vi "Slaver.vi"() -> ()   [LabVIEW 2014]
panel:
  out "에러 출력":errorcluster
  out "웨이브폼 그래프":dbl[](graph)
  in  "정지":bool
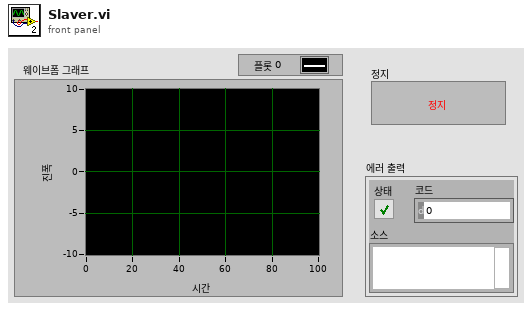
[diagram p1: front panel]
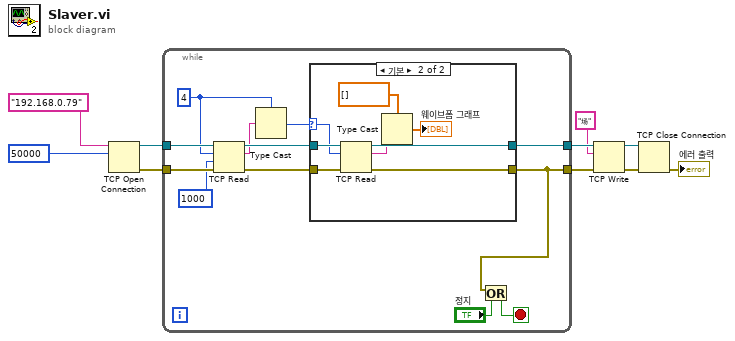
[diagram p0: block diagram]
diagram:
  n1 = TCP Open Connection(address="192.168.0.79" ("주소"), remote port or service name=u16 50000 ("원격 포트 또는 서비스 이름")) -> (connection ID=w8:refnum<k5>, error out=w7:errorcluster)  [unwired: 3 in]
  n2 = while {
    tunnel: w8 -> [w22]
    tunnel: [w20] -> w4
    tunnel: w7 -> [w19]
    tunnel: [w12] -> w3
    stop <- w13 stop-if-true
    w16 = 4 ("읽을 바이트")
    n3 = TCP Read(connection ID=w22, bytes to read=w16, error in (no error)=w19, 9:1000 ("타임아웃 ms (25000)")) -> (connection ID out=w21:refnum<k5>, data out=w17:string, error out=w15:errorcluster)  [unwired: 1 in]
    n4 = Type Cast(type=w16, x=w17) -> (*(type *) &x=w14:i32)
    n5 = case shown="기본" w14 {
      selector: w14 -> [_ w28]
      tunnel: w21 -> [w24 w32]
      tunnel: [w24 w31] -> w20
      tunnel: w15 -> [w23 w30]
      tunnel: [w23 w29] -> w12
      frame ..0 {
      }
      frame Default {
        n6 = TCP Read(connection ID=w32, bytes to read=w28, error in (no error)=w30) -> (connection ID out=w31:refnum<k5>, data out=w27:string, error out=w29:errorcluster)  [unwired: 2 in]
        n7 = Type Cast(type=dbl[] [] ("웨이브폼 그래프"), x=w27) -> (*(type *) &x=→"웨이브폼 그래프":dbl[])
      }
    }
    n8 = Or(x=w12, y="정지") -> (x .or. y?=w13:bool)
  }
  n9 = TCP Write(connection ID=w4, data in="场" ("데이터 입력"), error in (no error)=w3) -> (connection ID out=w5:refnum<k5>, error out=w6:errorcluster)  [unwired: 1 in, 1 out]
  n10 = TCP Close Connection(connection ID=w5, error in (no error)=w6) -> (error out=→"에러 출력":errorcluster)  [unwired: 1 in, 1 out]
